vi "RL_format.vi"(0 "R":dbl, 3 "X":dbl) -> (6 "R":string, 9 "L":string)   [LabVIEW 2020]
panel:
  in  "X? ou L":bool=TRUE
  in  "tamanho":i32=5
  out "length 2":i32
  out "length":i32
  # "FORMAT RL"
  # "6"
  # "12"
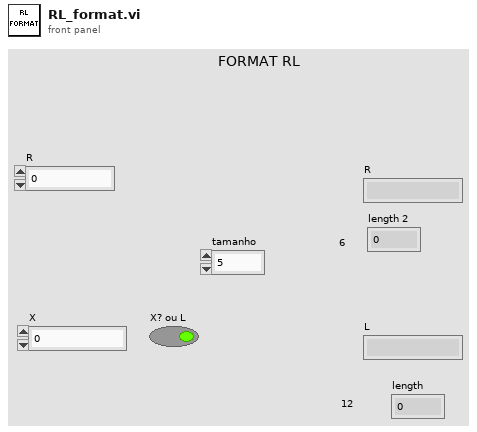
[diagram p1: front panel]
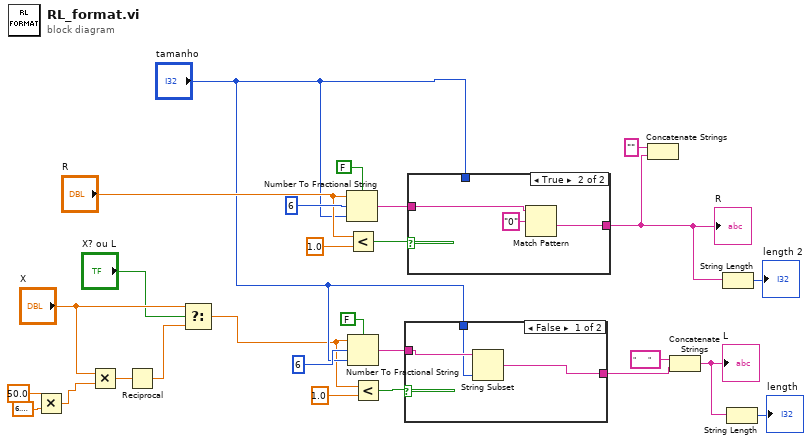
[diagram p0: block diagram]
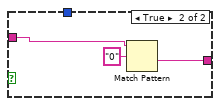
[diagram p2: hidden frame]
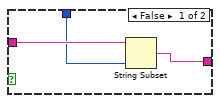
[diagram p3: hidden frame]
diagram:
  n1 = Multiply(x=50.0, y=6.283185307179586) -> (x*y=w12:dbl)
  n2 = Multiply(x="X", y=w12) -> (x*y=w11:dbl)
  n3 = Reciprocal(x=w11) -> (1/x=w3:dbl)
  n4 = Select(t="X", s="X? ou L", f=w3) -> (s? t:f=w5:dbl)
  n5 = Number To Fractional String(use system decimal point (T)=FALSE, number="R", width (-)=i16 6, precision (6)="tamanho") -> (F-format string=w21:string)
  n6 = Less?(x="R", y=1.0) -> (x < y?=w22:bool)
  n7 = Number To Fractional String(use system decimal point (T)=FALSE, number=w5, width (-)=i16 6, precision (6)="tamanho") -> (F-format string=w18:string)
  n8 = Less?(x=w5, y=1.0) -> (x < y?=w19:bool)
  n9 = case shown="False" w19 {
    tunnel: [w30 w32] -> w16
    tunnel: w18 -> [w29 w31]
    tunnel: "tamanho" -> [w28 _]
    frame False {
      n10 = String Subset(string=w29, length (rest)=w28) -> (substring=w30:string)  [unwired: 1 in]
    }
    frame True {
      n11 = Match Pattern(string=w31, regular expression="0") -> (after substring=w32:string)  [unwired: 1 in, 3 out]
    }
  }
  n12 = case shown="True" w22 {
    tunnel: w21 -> [w36 w38]
    tunnel: [w35 w37] -> w1
    tunnel: "tamanho" -> [w34 _]
    frame False {
      n13 = String Subset(string=w36, length (rest)=w34) -> (substring=w35:string)  [unwired: 1 in]
    }
    frame True {
      n14 = Match Pattern(string=w38, regular expression="0") -> (after substring=w37:string)  [unwired: 1 in, 3 out]
    }
  }
  "R" <- w1
  n15 = Concatenate Strings("" ("string"), w1) -> ()  [unwired: 1 out]
  n16 = Concatenate Strings("      " ("string"), w16) -> (w10:string)
  "L" <- w10
  n17 = String Length(string=w1) -> (length=→"length 2":i32)
  n18 = String Length(string=w10) -> (length=→"length":i32)
